vi "Read Lines From File (with error IO).vi"(0 "file path (dialog if empty)":path, 5 "number of rows (all:-1)":i32=-1, 7 "convert eol? (F)":bool, 11 "error in (no error)":errorcluster, 12 "start of read offset (chars.:0)":i32, 13 "max characters/row  (no limit:0)":i32) -> (4 "new file path (Not A Path if cancelled)":path, 6 "line string":string, 8 "mark after read (chars.)":i32, 10 "EOF?":bool, 15 "error out":errorcluster)   [LabVIEW 2020]
doc: "Reads a specified number of lines from a byte stream file beginning at a specified character offset. The VI opens the file before reading from it and closes it afterwards."
panel:
  in  "prompt":string="Choose file to read."
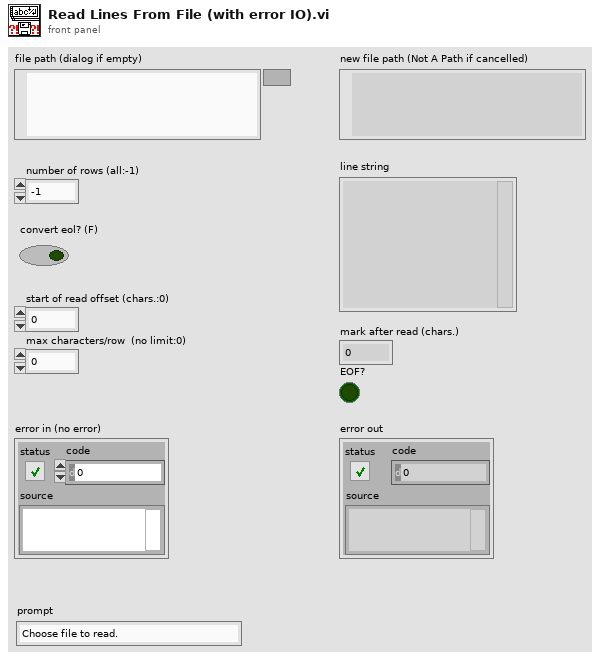
[diagram p1: front panel]
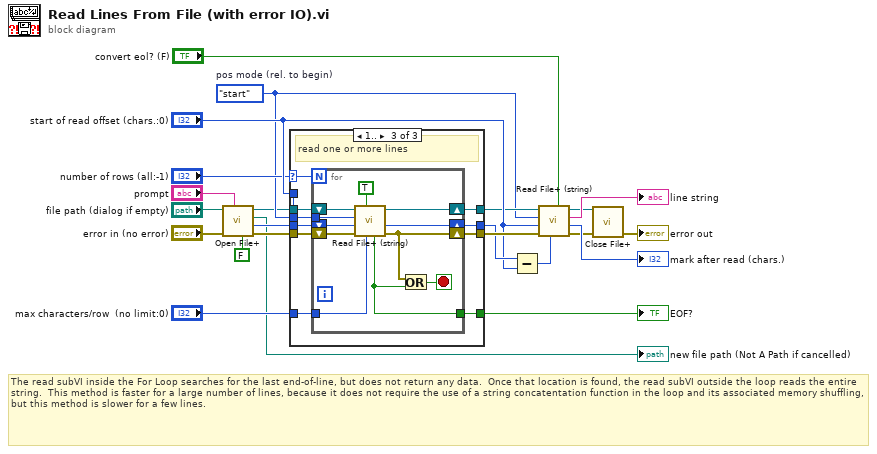
[diagram p0: block diagram]
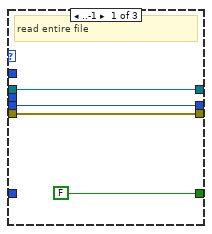
[diagram p2: hidden frame]
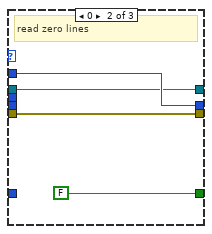
[diagram p3: hidden frame]
diagram:
  w13 = enum16{"start", "end", "current"}."start"  # pos mode (rel. to begin)
  # "The read subVI inside the For Loop searches for the last end-of-line, but does not return any data.  Once that location is found, the read subVI outside the loop reads the entire string.  This method is faster for a large number of lines, because it does not require the use of a string concatentation function in the loop and its associated memory shuffling, but this method is slower for a few lines."
  n1 = call "Open File+.vi"("advisory dialog? (display:T)"=FALSE, "prompt"="prompt", "error in (not an error)"="error in (no error)", "file path (\" \")"="file path (dialog if empty)") -> ("error out"=w12:errorcluster, "file size (bytes)"=w11:i32, "file path"=→"new file path (Not A Path if cancelled)":path, "refnum"=w9:refnum<file>)  [unwired: 4 in]
  n2 = case shown="1.." "number of rows (all:-1)" {
    selector: "number of rows (all:-1)" -> [_ _ w32]
    tunnel: [w27 w30 w41] -> w20
    tunnel: [w26 w31 w40] -> w19
    tunnel: "max characters/row  (no limit:0)" -> [_ _ w39]
    tunnel: w12 -> [w27 w30 w38]
    tunnel: w9 -> [w25 w29 w37]
    tunnel: "start of read offset (chars.:0)" -> [_ w31 w36]
    tunnel: w13 -> [_ _ w35]
    tunnel: w11 -> [w26 _ _]
    tunnel: [w25 w29 w34] -> w16
    tunnel: [FALSE FALSE w33] -> w15
    frame ..-1 {
      # "read entire file"
    }
    frame 0 {
      # "read zero lines"
    }
    frame 1.. {
      # "read one or more lines"
      n3 = for {
        N: w32 -> [_]
        tunnel: [w44] -> w33
        tunnel: w35 -> [w46]
        tunnel: w39 -> [w48]
        shift-left: w36 -> [w51]
        shift-right: [w52] -> w40
        shift-right: [w43] -> w41
        shift-left: w38 -> [w47]
        shift-right: [w50] -> w34
        shift-left: w37 -> [w49]
        stop <- w42 stop-if-true
        n4 = call "Read File+ (string).vi"("count"=w48, "line mode (characters:F)"=TRUE ("read line"), "error in (no error)"=w47, "pos offset (bytes:0)"=w51, "pos mode (rel. to current:2)"=w46, "refnum"=w49) -> ("error out"=w43:errorcluster, "mark after read (bytes)"=w52:i32, "dup refnum"=w50:refnum<file>, "EOF?"=w44:bool)  [unwired: 1 in, 1 out]
        n5 = Or(x=w43, y=w44) -> (x .or. y?=w42:bool)
      }
    }
  }
  "EOF?" <- w15
  n6 = Subtract(x=w19, y="start of read offset (chars.:0)") -> (x-y=w23:i32)
  n7 = call "Read File+ (string).vi"("convert eol? (no:F)"="convert eol? (F)", "count"=w23, "error in (no error)"=w20, "pos offset (bytes:0)"="start of read offset (chars.:0)", "pos mode (rel. to current:2)"=w13, "refnum"=w16) -> ("error out"=w6:errorcluster, "mark after read (bytes)"=→"mark after read (chars.)":i32, "string"=→"line string":string, "dup refnum"=w4:refnum<file>)  [unwired: 1 in, 1 out]
  n8 = call "Close File+.vi"("error in (no error)"=w6, "refnum"=w4) -> ("error out"=→"error out":errorcluster)  [unwired: 3 in, 2 out]
